vi "Convert Engine to String.vi"(7 "transfer group id":i32, 8 "error in":errorcluster, 9 "string buffer":refnum<class "Buffer.lvclass">, 10 "engine buffer":refnum<class "Buffer.lvclass">, 11 "DSF buffer converter in":refnum<class "Default Buffer Converter.lvclass">) -> (0 "error out":errorcluster, 3 "DSF buffer converter out":refnum<class "Default Buffer Converter.lvclass">)   [LabVIEW 2021, in "DSF Core.lvlib" / "Default Buffer Converter.lvclass"]
uses:
  Default Buffer Converter.lvclass
  Classes/Buffer/Buffer.lvclass
  C:/Program Files/National Instruments/LabVIEW 2021/vi.lib/NI/Memory Manager/Classes/Pointer/Pointer.lvclass
  Default Buffer Converter.lvclass/Default Buffer Converter.ctl
  <vilib>/NI/Memory Manager/Classes/Pointer/Pointer.lvclass/Pointer.ctl
  <vilib>/NI/Memory Manager/Classes/Pointer/Write.vi
  <vilib>/NI/Memory Manager/Classes/Pointer/Write 1D U8.vi
  <vilib>/NI/Memory Manager/Classes/Pointer/Read.vi
  <vilib>/NI/Memory Manager/Classes/Pointer/Read 1D U8.vi
  <vilib>/NI/Memory Manager/Classes/Pointer/Write (No Check).vi
  <vilib>/NI/Memory Manager/Classes/Pointer/Write (No Check) 1D U8.vi
  <vilib>/NI/Memory Manager/Classes/Pointer/Check Move.vi
  <vilib>/NI/Memory Manager/Classes/Pointer/Read (No Check).vi
  <vilib>/NI/Memory Manager/Classes/Pointer/Read (No Check) 1D U8.vi
  <vilib>/NI/Memory Manager/Classes/Pointer/Get Address.vi
  <vilib>/NI/Memory Manager/Classes/Pointer/Check Null Pointer.vi
  <vilib>/NI/Memory Manager/Classes/Pointer/Check Count.vi
  <vilib>/NI/Memory Manager/Classes/Pointer/Check Bounds (Power of 2).vi
  <vilib>/NI/Memory Manager/Classes/Pointer/Errors.vi
  <vilib>/NI/Memory Manager/Classes/Pointer/Null Pointer.vi
  <vilib>/NI/Memory Manager/Classes/Pointer/Is Null.vi
  <vilib>/NI/Memory Manager/Classes/Pointer/Get Size.vi
  <vilib>/NI/Memory Manager/Classes/Pointer/Out of Bounds.vi
  <vilib>/NI/Memory Manager/Classes/Pointer/Check Bounds.vi
  <vilib>/NI/Memory Manager/Classes/Pointer/Create Error.vi
  <vilib>/NI/Memory Manager/VIs/Write String to Source.vi
  <vilib>/NI/Memory Manager/Classes/Pointer/Write Pointer Size to Error.vi
  <vilib>/NI/Memory Manager/VIs/Write Numeric to Source.vi
  <vilib>/NI/Memory Manager/VIs/Write Numeric Scalar to Source (Base10 U64).vi
  <vilib>/NI/Memory Manager/Classes/Pointer/Check Bounds (Pointer).vi
  <vilib>/NI/Memory Manager/Classes/Pointer/Check Bounds (Buffer).vi
  <vilib>/NI/Memory Manager/VIs/New Error Cluster.vi
  <vilib>/NI/Memory Manager/VIs/New Error Cluster (512B).vi
  <vilib>/NI/Memory Manager/VIs/Set Error Status.vi
  <vilib>/NI/Memory Manager/VIs/Set Error Code.vi
  <vilib>/NI/Memory Manager/VIs/Set Error Source.vi
  <vilib>/NI/Memory Manager/Constants/Constants.vi
  <vilib>/NI/Memory Manager/Constants/Library Name.vi
  <vilib>/NI/Memory Manager/Classes/Pointer/Pointer Error Info.vi
  <vilib>/NI/Memory Manager/Constants/Pointer Class Name.vi
  <vilib>/NI/Memory Manager/Classes/Pointer/Buffer Underflow.vi
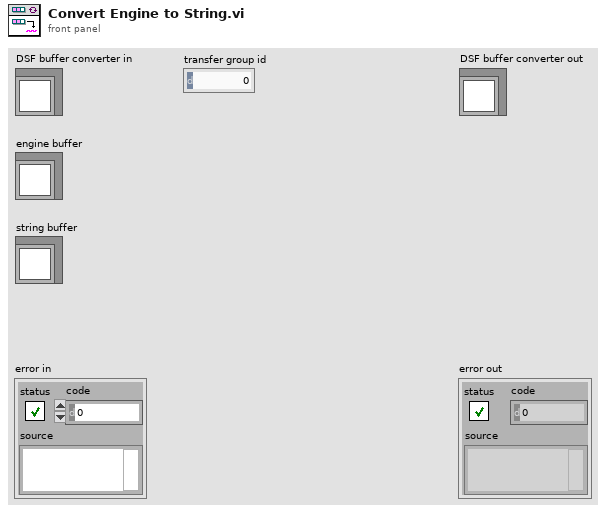
[diagram p1: front panel]
types:
  T1 = typedef "DSF Core.lvlib/Default Buffer Converter.lvclass/Conversion.ctl" = cluster{"conversion blocks":T2[]}
  T2 = typedef "DSF Core.lvlib/Default Buffer Converter.lvclass/Conversion Block.ctl" = cluster{"engine offset":u64, "engine data type":T3, "string offset":u64, "string data type":T3, "engine byte order":enum16{"big-endian, network order", "native, host order", "little-endian"}, "string byte order":enum16{"big-endian, network order", "native, host order", "little-endian"}, "count":u64}
  T3 = typedef "DSF Core.lvlib/DSF Data Type.ctl" = enum8{"Bool", "SGL", "DBL", "I8", "I16", "I32", "I64", "U8", "U16", "U32", "U64"}
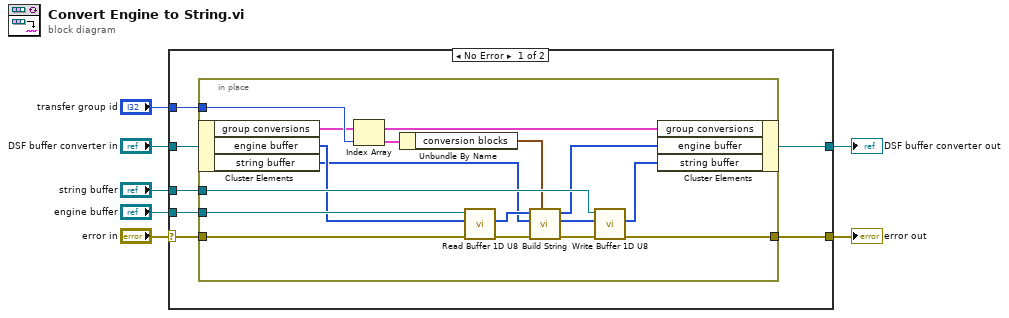
[diagram p0: block diagram]
diagram:
  n1 = case shown="No Error" "error in" {
    selector: "error in" -> [w11 w32]
    tunnel: [w10 w32] -> w6
    tunnel: [w8 w31] -> w4
    tunnel: "DSF buffer converter in" -> [w9 w31]
    tunnel: "transfer group id" -> [w14 _]
    tunnel: "engine buffer" -> [w13 _]
    tunnel: "string buffer" -> [w12 _]
    frame No Error {
      n2 = in-place {
        in-place-border: w14 -> [w29]
        in-place-border: w13 -> [w25]
        in-place-border: w12 -> [w24]
        in-place-border: w11 -> [w22]
        in-place-border: [w21] -> w10
        n3 = in-place-cluster #1(w9) -> ("group conversions"=w15:T1[], "engine buffer"=w19:u8[], "string buffer"=w18:u8[])
        n4 = Index Array(array=w15, index=w29) -> (element=w30:T1)
        n5 = Unbundle By Name(w30) -> ("conversion blocks"=w20:T2[])
        n6 = call "Read Buffer 1D U8.vi"("error in (no error)"=w22, "dst array in"=w19, "Buffer in"=w25) -> ("error out"=w28:errorcluster, "dst array out"=w26:u8[])  [unwired: 5 in, 2 out]
        n7 = call "Build String.vi"("conversion blocks"=w20, "error in (no error)"=w28, "string buffer in"=w18, "engine buffer in"=w26) -> ("error out"=w27:errorcluster, "string buffer out"=w23:u8[], "engine buffer out"=w16:u8[])  [unwired: 5 in]
        n8 = call "Write Buffer 1D U8.vi"("error in (no error)"=w27, "src array in"=w23, "Buffer in"=w24) -> ("error out"=w21:errorcluster, "src array out"=w17:u8[])  [unwired: 5 in, 2 out]
        n9 = in-place-cluster #1("group conversions"=w15, "engine buffer"=w16, "string buffer"=w17) -> (w8:refnum<class "Default Buffer Converter.lvclass">)
      }
    }
    frame Error {
    }
  }
  "error out" <- w6
  "DSF buffer converter out" <- w4
